vi "Vision Processing.vi"(4 "error in (no error)":errorcluster, 7 "Image Size":T1=enum."320x240") -> ()   [LabVIEW 2013]
doc: "This VI runs in parallel to other tasks. It gets images from the camera, processes them for color or shape and use that information to affect robot behavior."
uses:
  <vilib>/Rock Robotics/WPI/Camera/WPI_CameraImageSize.ctl
  <vilib>/Rock Robotics/WPI/Camera/WPI_CameraWhite Balance Values.ctl
  <vilib>/Rock Robotics/WPI/Camera/WPI_CameraExposure Values.ctl
  <vilib>/Rock Robotics/WPI/Camera/WPI_CameraFrameRate.ctl
  Robot Global Data.vi
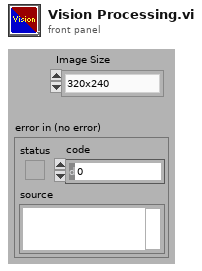
[diagram p1: front panel]
types:
  T1 = typedef "WPI_CameraImageSize.ctl" = enum16{"640x480", "320x240", "160x120"}
  T2 = typedef "WPI_CameraFrameRate.ctl" = u32
  T3 = typedef "WPI_CameraExposure Values.ctl" = enum16{"Auto", "Flicker-free 50 Hz", "Flicker-free 60 Hz", "Hold current"}
  T4 = typedef "WPI_CameraWhite Balance Values.ctl" = enum16{"Auto", "Fixed indoor", "Fixed outdoor 1", "Fixed outdoor 2", "Fixed fluorescent 1", "Fixed fluorescent 2", "Hold current"}
  T5 = typedef "Image Type" = u32
  T6 = typedef "WPI_CameraDevRef.ctl" = cluster{"Camera Address":string, "CameraStatus":errorcluster, "Acquire Image Notifier":refnum<notifier>}
  T7 = typedef "IMAQ Image.ctl" = refnum<image>
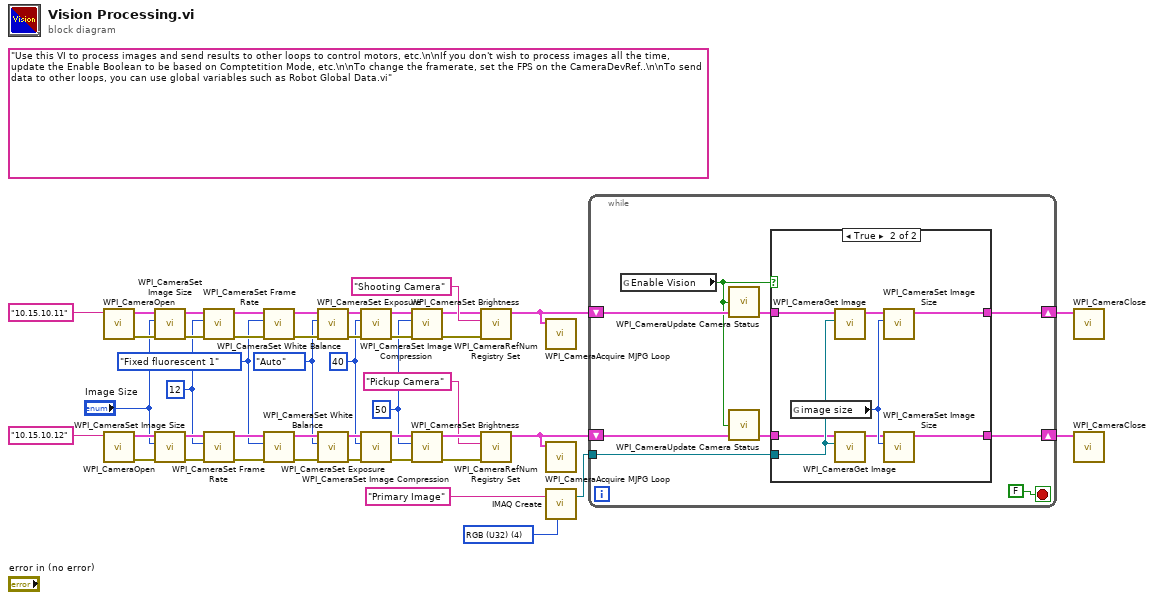
[diagram p0: block diagram]
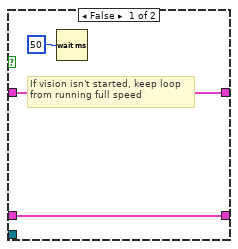
[diagram p2: hidden frame]
diagram:
  w5 = T2 12 ("Frame Rate (fps)")
  w3 = WPI_CameraExposure_Values."Auto" ("Exposure")
  w4 = WPI_CameraWhite_Balance_Values."Fixed fluorescent 1" ("White Balance")
  w1 = 50 ("Brightness")
  w2 = 40 ("Compression")
  (unwired) "Use this VI to process images and send results to other loops to control motors, etc.\n\nIf you don't wish to process images all the time, update the Enable Boolean to be based on Comptetition Mode, etc.\n\nTo change the framerate, set the FPS on the CameraDevRef..\n\nTo send data to other loops, you can use global variables such as Robot Global Data.vi"
  w45 = T5 4 items=["Grayscale (U8)", "Grayscale (I16)", "Grayscale (SGL)", "Complex (CSG)", "RGB (U32)", "HSL (U32)", "RGB (U64)"] ("Image Type")
  n1 = call <vilib>:"WPI_CameraOpen.vi"("Camera Address"="10.15.10.11") -> ("error out"=w35:errorcluster, "CameraDevRef"=w36:T6)  [unwired: 1 in, 8 out]
  n2 = call <vilib>:"WPI_CameraOpen.vi"("Camera Address"="10.15.10.12") -> ("error out"=w18:errorcluster, "CameraDevRef"=w17:T6)  [unwired: 1 in, 8 out]
  n3 = call <vilib>:"WPI_CameraSet Image Size.vi"("error in (no error)"=w35, "Image Size"="Image Size", "CameraDevRef"=w36) -> ("error out"=w34:errorcluster, "CameraDevRef Out"=w37:T6)  [unwired: 7 out]
  n4 = call <vilib>:"WPI_CameraSet Image Size.vi"("error in (no error)"=w18, "Image Size"="Image Size", "CameraDevRef"=w17) -> ("error out"=w19:errorcluster, "CameraDevRef Out"=w16:T6)  [unwired: 7 out]
  n5 = call <vilib>:"WPI_CameraSet Frame Rate.vi"("error in (no error)"=w34, "Frame Rate (fps)"=w5, "CameraDevRef"=w37) -> ("error out"=w33:errorcluster, "CameraDevRef Out"=w39:T6)  [unwired: 7 out]
  n6 = call <vilib>:"WPI_CameraSet Frame Rate.vi"("error in (no error)"=w19, "Frame Rate (fps)"=w5, "CameraDevRef"=w16) -> ("error out"=w20:errorcluster, "CameraDevRef Out"=w14:T6)  [unwired: 7 out]
  n7 = call <vilib>:"WPI_CameraSet White Balance.vi"("error in (no error)"=w33, "White Balance"=w4, "CameraDevRef"=w39) -> ("error out"=w32:errorcluster, "CameraDevRef Out"=w38:T6)  [unwired: 7 out]
  n8 = call <vilib>:"WPI_CameraSet White Balance.vi"("error in (no error)"=w20, "White Balance"=w4, "CameraDevRef"=w14) -> ("error out"=w21:errorcluster, "CameraDevRef Out"=w15:T6)  [unwired: 7 out]
  n9 = call <vilib>:"WPI_CameraSet Exposure.vi"("error in (no error)"=w32, "Exposure"=w3, "CameraDevRef"=w38) -> ("error out"=w31:errorcluster, "CameraDevRef Out"=w41:T6)  [unwired: 7 out]
  n10 = call <vilib>:"WPI_CameraSet Exposure.vi"("error in (no error)"=w21, "Exposure"=w3, "CameraDevRef"=w15) -> ("error out"=w22:errorcluster, "CameraDevRef Out"=w12:T6)  [unwired: 7 out]
  n11 = call <vilib>:"WPI_CameraSet Image Compression.vi"("error in (no error)"=w31, "Compression"=w2, "CameraDevRef"=w41) -> ("error out"=w30:errorcluster, "CameraDevRef Out"=w40:T6)  [unwired: 7 out]
  n12 = call <vilib>:"WPI_CameraSet Image Compression.vi"("error in (no error)"=w22, "Compression"=w2, "CameraDevRef"=w12) -> ("error out"=w23:errorcluster, "CameraDevRef Out"=w13:T6)  [unwired: 7 out]
  n13 = call <vilib>:"WPI_CameraSet Brightness.vi"("error in (no error)"=w30, "Brightness"=w1, "CameraDevRef"=w40) -> ("error out"=w28:errorcluster, "CameraDevRef Out"=w29:T6)  [unwired: 7 out]
  n14 = call <vilib>:"WPI_CameraSet Brightness.vi"("error in (no error)"=w23, "Brightness"=w1, "CameraDevRef"=w13) -> ("error out"=w25:errorcluster, "CameraDevRef Out"=w24:T6)  [unwired: 7 out]
  n15 = call <vilib>:"WPI_CameraRefNum Registry Set.vi"("error in (no error)"=w28, "refnum name"="Shooting Camera", "CameraDevRef"=w29) -> ("CameraDevRef"=w27:T6)  [unwired: 8 out]
  n16 = call <vilib>:"WPI_CameraRefNum Registry Set.vi"("error in (no error)"=w25, "refnum name"="Pickup Camera", "CameraDevRef"=w24) -> ("CameraDevRef"=w10:T6)  [unwired: 8 out]
  n17 = call <vilib>:"WPI_CameraAcquire MJPG Loop.vi"("CameraDevRef"=w27) -> ()  [unwired: 11 in]
  n18 = call <vilib>:"WPI_CameraAcquire MJPG Loop.vi"("CameraDevRef"=w10) -> ()  [unwired: 11 in]
  n19 = call "IMAQ Create"("Image Name"="Primary Image", "Image Type"=w45) -> ("New Image"=w43:T7)  [unwired: 2 in, 2 out]
  n20 = while {
    shift-right: [w53] -> w26
    shift-left: w27 -> [w51]
    tunnel: w43 -> [w52]
    shift-right: [w47] -> w9
    shift-left: w10 -> [w46]
    stop <- FALSE stop-if-true
    n21 = global read "Robot Global Data.vi" "Enable Vision"() -> (w49:bool)
    n22 = call <vilib>:"WPI_CameraUpdate Camera Status.vi"("CameraDevRef In"=w51, "Enable Vision"=w49) -> ("CameraDevRef Out"=w50:T6)  [unwired: 3 in]
    n23 = call <vilib>:"WPI_CameraUpdate Camera Status.vi"("CameraDevRef In"=w46, "Enable Vision"=w49) -> ("CameraDevRef Out"=w48:T6)  [unwired: 3 in]
    n24 = case shown="True" w49 {
      tunnel: w52 -> [_ w62]
      tunnel: [w57 w65] -> w53
      tunnel: w50 -> [w57 w64]
      tunnel: w48 -> [w55 w61]
      tunnel: [w55 w58] -> w47
      frame False {
        # "If vision isn't started, keep loop\nfrom running full speed"
        n25 = Wait (ms)(milliseconds to wait=u32 50) -> ()  [unwired: 1 out]
      }
      frame True {
        n26 = global read "Robot Global Data.vi" "image size"() -> (w60:T1)
        n27 = call <vilib>:"WPI_CameraGet Image.vi"("Image"=w62, "CameraDevRef"=w64) -> ("CameraDevRef Out"=w63:T6)  [unwired: 1 in, 8 out]
        n28 = call <vilib>:"WPI_CameraGet Image.vi"("Image"=w62, "CameraDevRef"=w61) -> ("CameraDevRef Out"=w59:T6)  [unwired: 1 in, 8 out]
        n29 = call <vilib>:"WPI_CameraSet Image Size.vi"("Image Size"=w60, "CameraDevRef"=w63) -> ("CameraDevRef Out"=w65:T6)  [unwired: 1 in, 8 out]
        n30 = call <vilib>:"WPI_CameraSet Image Size.vi"("Image Size"=w60, "CameraDevRef"=w59) -> ("CameraDevRef Out"=w58:T6)  [unwired: 1 in, 8 out]
      }
    }
  }
  n31 = call <vilib>:"WPI_CameraClose.vi"("CameraDevRef"=w26) -> ()  [unwired: 1 in, 10 out]
  n32 = call <vilib>:"WPI_CameraClose.vi"("CameraDevRef"=w9) -> ()  [unwired: 1 in, 10 out]
